vi "190613_mesin.vi"() -> ()   [LabVIEW 2017]
uses:
  <vilib>/Instr/_visa.llb/VISA Configure Serial Port (Instr).vi
panel:
  out "Jam Login":string
  out "String mesin":string
  in  "COM Port":refnum<visa-resource-name>
  out "Status Mesin":bool
  out "String P4":string
  out "P4":bool
  out "String P3":string
  out "P3":bool
  out "String P2":string
  out "P2":bool
  out "String P1":string
  out "Nama":string
  out "ID":string
  out "P1":bool
  out "dara received":string
  out "RPM":dbl(knob) scale=0.0..500.0
  in  "stop":bool
  out "error out":errorcluster
  # "SISTEM AKUISISI DATA MESIN PENGGULUNG KABEL \nDENGAN AUTENTIFIKASI OPERATOR MENGGUNAKAN RFID"
  # "Neni Elyawati\nNRP 10311600010041"
  # "Identitas Pengguna"
  # "Com Port"
  # "Status Mesin"
  # "Kecepatan Motor"
  # "RPM"
  # "Status Sensor"
  # "Sensor Batas Kanan"
  # "Sensor Kabel Tegang"
  # "Sensor Kabel Kendor"
  # "Sensor Batas Kiri"
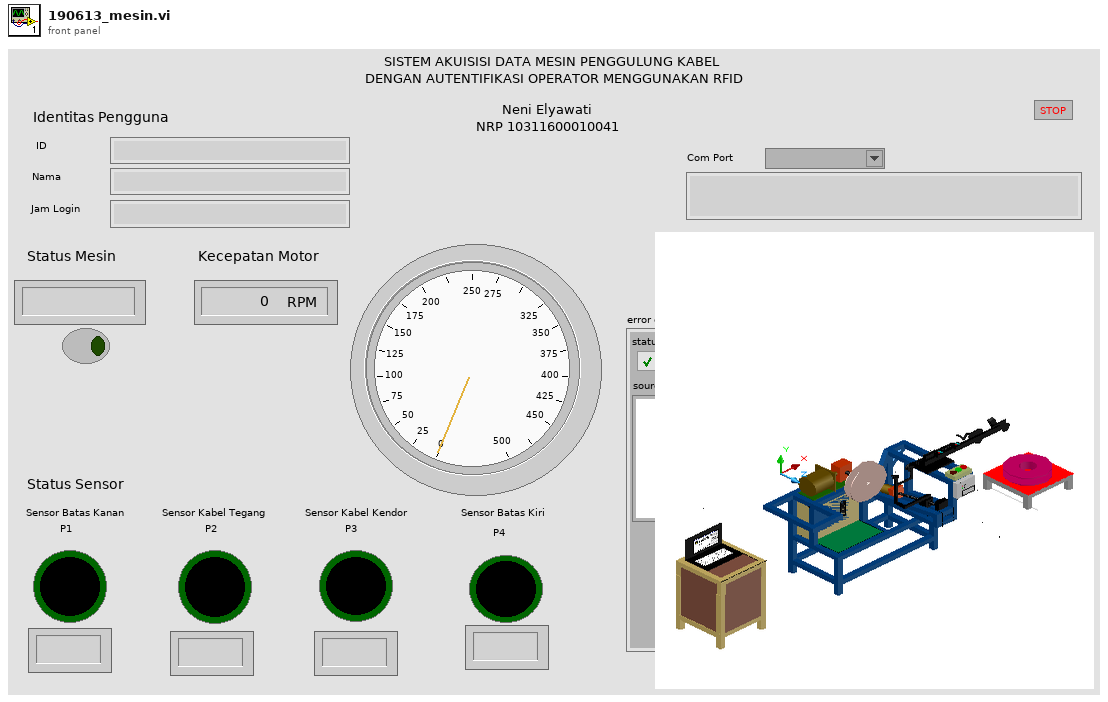
[diagram p1: front panel]
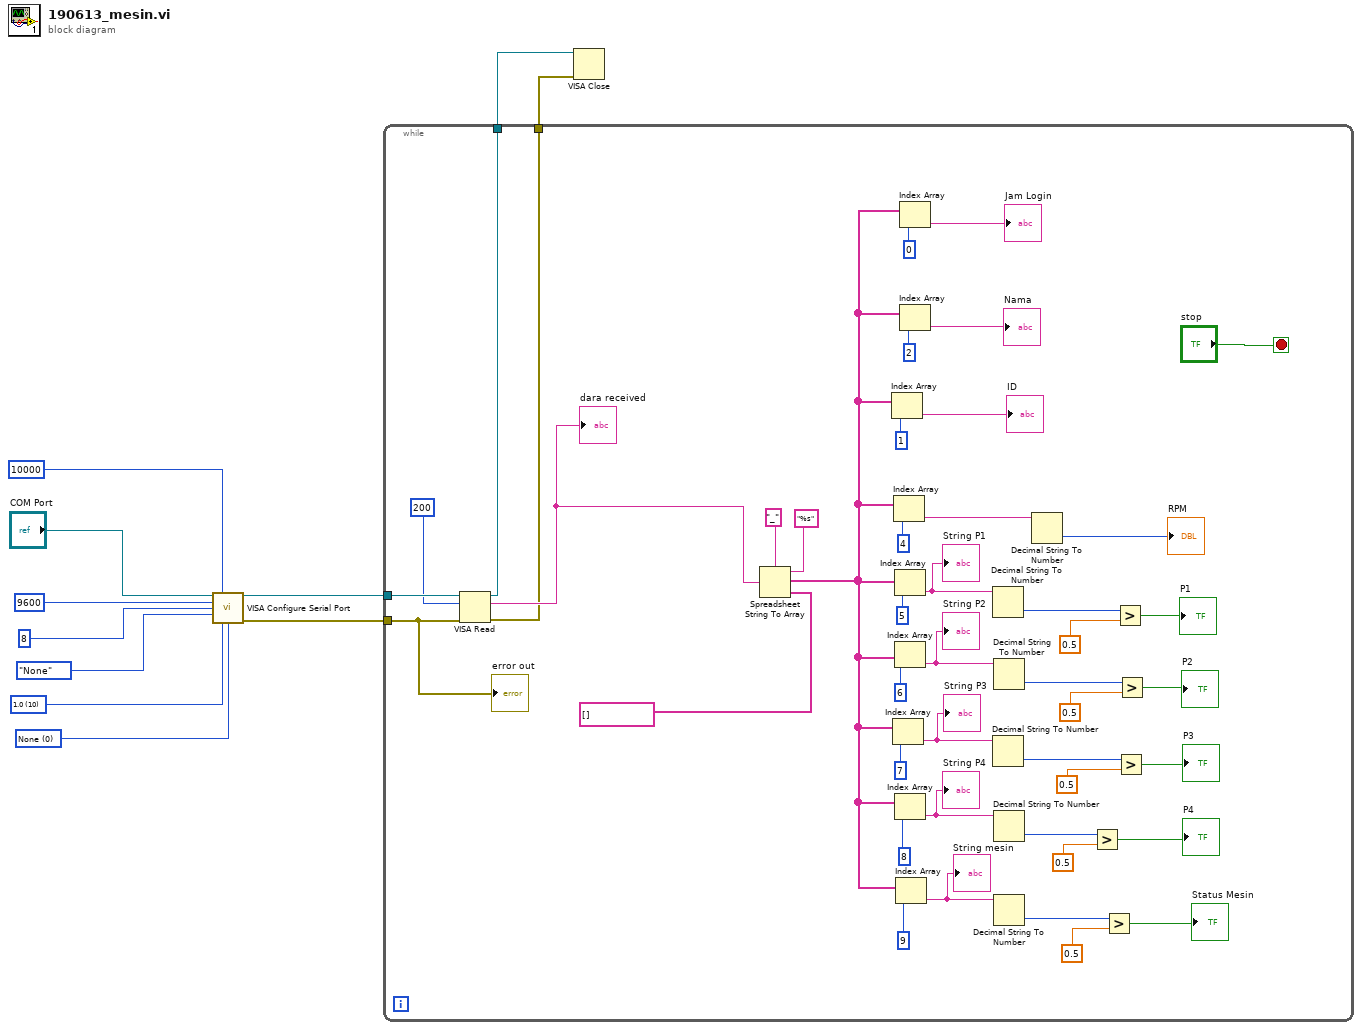
[diagram p0: block diagram]
diagram:
  w6 = u16 10 items=["1.0"=10, "1.5"=15, "2.0"=20] ("stop bits (10: 1 bit)")
  w5 = u16 0 items=["None", "XON/XOFF", "RTS/CTS", "XON/XOFF & RTS/CTS", "DTR/DSR", "XON/XOFF & DTR/DSR"] ("flow control (0:none)")
  n1 = call-poly "VISA Configure Serial Port"("VISA resource name"="COM Port", "timeout (10sec)"=u32 10000, "baud rate (9600)"=u32 9600, "data bits (8)"=u16 8, "parity (0:none)"=enum16{"None", "Odd", "Even", "Mark", "Space"}."None", "stop bits (10: 1 bit)"=w6, "flow control (0:none)"=w5) -> ("VISA resource name out"=w4:refnum<visa-resource-name>, "error out"=w1:errorcluster)  [unwired: 7 in]
  n2 = while {
    tunnel: w4 -> [w42]
    tunnel: [w40] -> w3
    tunnel: [w39] -> w2
    tunnel: w1 -> [w38]
    stop <- "stop" stop-if-true
    n3 = VISA Read(VISA resource name=w42, byte count=u32 200, error in (no error)=w38) -> (VISA resource name out=w39:refnum<visa-resource-name>, read buffer=w43:string, error out=w40:errorcluster)  [unwired: 1 out]
    "dara received" <- w43
    n4 = Spreadsheet String To Array(delimiter (Tab)="_", format string="%s", spreadsheet string=w43, array type (2D Dbl)=string[] []) -> (array=w23:string[])
    n5 = Index Array(array=w23, index=1) -> (element=→"ID":string)
    n6 = Index Array(array=w23, index=7) -> (element=w14:string)
    "String P3" <- w14
    n7 = Index Array(array=w23, index=4) -> (element=w35:string)
    n8 = Index Array(array=w23, index=5) -> (element=w12:string)
    "String P1" <- w12
    n9 = Index Array(array=w23, index=6) -> (element=w13:string)
    "String P2" <- w13
    n10 = Index Array(array=w23, index=8) -> (element=w15:string)
    "String P4" <- w15
    n11 = Index Array(array=w23, index=9) -> (element=w16:string)
    "String mesin" <- w16
    n12 = Index Array "Index Array"(array=w23, index=0) -> (element=→"Jam Login":string)
    n13 = Index Array "Index Array"(array=w23, index=2) -> (element=→"Nama":string)
    n14 = Decimal String To Number(string=w12) -> (number=w33:i32)  [unwired: 2 in, 1 out]
    n15 = Decimal String To Number(string=w14) -> (number=w31:i32)  [unwired: 2 in, 1 out]
    n16 = Decimal String To Number(string=w13) -> (number=w32:i32)  [unwired: 2 in, 1 out]
    n17 = Decimal String To Number(string=w15) -> (number=w30:i32)  [unwired: 2 in, 1 out]
    n18 = Decimal String To Number(string=w16) -> (number=w29:i32)  [unwired: 2 in, 1 out]
    n19 = Decimal String To Number(string=w35) -> (number=→"RPM":i32)  [unwired: 2 in, 1 out]
    n20 = Greater?(x=w30, y=0.5) -> (0:→"P4":bool)
    n21 = Greater?(x=w29, y=0.5) -> (0:→"Status Mesin":bool)
    n22 = Greater?(x=w33, y=0.5) -> (0:→"P1":bool)
    n23 = Greater?(x=w31, y=0.5) -> (0:→"P3":bool)
    n24 = Greater?(x=w32, y=0.5) -> (0:→"P2":bool)
    "error out" <- w38
  }
  n25 = VISA Close(VISA resource name=w2, error in (no error)=w3) -> ()  [unwired: 1 out]
